vi "SetGraphAttribute.vi"(8 "error in":errorcluster caption="错误输入（无错误）", 9 "Display Mode":T1, 10 "CH Tag[]":string[](array[string]), 11 "波形图表":refnum<vi>) -> (0 "error out":errorcluster caption="错误输出")   [LabVIEW 2016]
uses:
  Display Mode.ctl
  PCM PanelSplit.lvclass
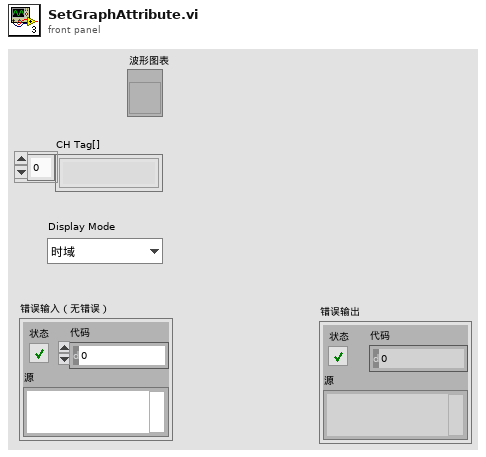
[diagram p1: front panel]
types:
  T1 = typedef "PCM PanelSplit.lvclass/Display Mode.ctl" = enum16{"时域", "频谱", "功率谱"}
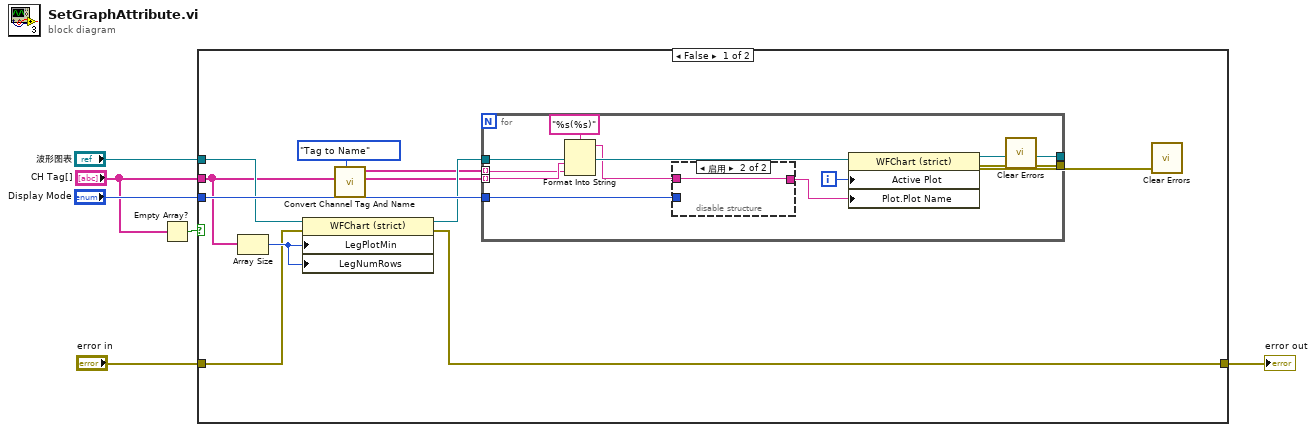
[diagram p0: block diagram]
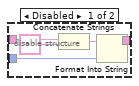
[diagram p2: hidden frame]
diagram:
  n1 = Empty Array?(array="CH Tag[]") -> (empty?=w3:bool)
  n2 = case shown="False" w3 {
    tunnel: "Display Mode" -> [w17 _]
    tunnel: "波形图表" -> [w15 _]
    tunnel: "CH Tag[]" -> [w9 _]
    tunnel: "error in" -> [w13 w35]
    tunnel: [w12 w35] -> w1
    frame False {
      n3 = Array Size(array=w9) -> (size(s)=w16:i32)
      n4 = property on="属性节点" class="WFChart (strict)"(reference=w15, error in=w13, "LegPlotMin"=w16, "LegNumRows"=w16) -> (reference out=w14:refnum<vi>, error out=w12:errorcluster)
      n5 = call "Convert Channel Tag And Name.vi"("Direction"=enum16{"Tag to Name", "Name to Tag"}."Tag to Name", "String[] in"=w9) -> ("String[] out"=w8:string[], "Unit[]"=w7:string[])  [unwired: 8 in]
      n6 = for {
        tunnel: w14 -> [w28]
        tunnel: w8 -> [w21] mode=indexing
        tunnel: w17 -> [w26]
        tunnel: [w23] -> w11
        tunnel: [w22] -> _
        tunnel: w7 -> [w20] mode=indexing
        i -> [w27]
        n7 = Format Into String(format string="%s(%s)" ("格式字符串"), w21, w20) -> (resulting string=w18:string)  [unwired: 2 in, 1 out]
        n8 = disable-structure shown="启用" {
          disable-tunnel: w26 -> [w33 _]
          disable-tunnel: [w32 w34] -> w25
          disable-tunnel: w18 -> [w30 w34]
          frame Disabled {
            n9 = Concatenate Strings(w30, " - " ("格式字符串")) -> (w31:string)
            n10 = Format Into String(initial string=w31, w33) -> (resulting string=w32:string)  [unwired: 2 in, 1 out]
          }
          frame Enabled {
          }
        }
        n11 = property class="WFChart (strict)"(reference=w28, "Active Plot"=w27, "Plot.Plot Name"=w25) -> (reference out=w22:refnum<vi>, error out=w24:errorcluster)  [unwired: 1 in]
        n12 = call <vilib>:"Clear Errors.vi"("error in (no error)"=w24) -> ("error out"=w23:errorcluster)  [unwired: 5 in, 1 out]
      }
      n13 = call <vilib>:"Clear Errors.vi"("error in (no error)"=w11) -> ()  [unwired: 5 in, 2 out]
    }
    frame True {
    }
  }
  "error out" <- w1
